vi "AppendToArray.vi"(5 "InputArray":dbl[](array[numeric]), 9 "Element":dbl, 11 "MaxArraySize":dbl) -> (8 "OutputArray":dbl[](array[numeric]))   [LabVIEW 2020]
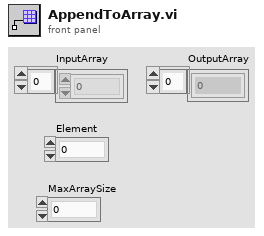
[diagram p1: front panel]
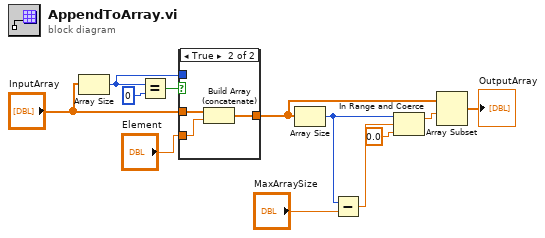
[diagram p0: block diagram]
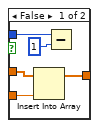
[diagram p2: hidden frame]
diagram:
  n1 = Array Size(array="InputArray") -> (size(s)=w8:i32)
  n2 = Equal?(x=w8, y=0) -> (x = y?=w10:bool)
  n3 = case shown="True" w10 {
    tunnel: "Element" -> [w16 w19]
    tunnel: "InputArray" -> [w17 w20]
    tunnel: [w13 w18] -> w7
    tunnel: w8 -> [w15 _]
    frame False {
      n4 = Insert Into Array(array=w17, new element=w16) -> (w13:dbl[])  [unwired: 1 in]
      n5 = Subtract(x=w15, y=1) -> ()  [unwired: 1 out]
    }
    frame True {
      n6 = Build Array (concatenate)(w20, w19) -> (w18:dbl[])
    }
  }
  n7 = Array Size(array=w7) -> (size(s)=w3:i32)
  n8 = Subtract(x=w3, y="MaxArraySize") -> (x-y=w4:dbl)
  n9 = In Range and Coerce(upper limit=w3, x=w4, lower limit=0.0) -> (coerced(x)=w1:dbl)  [unwired: 1 out]
  n10 = Array Subset(array=w7, index=w1) -> (→"OutputArray":dbl[])  [unwired: 1 in]
